vi "Change Panel.vi"(8 "error in (no error)":errorcluster, 10 "New Panel":refnum<class "Panel.lvclass">, 11 "Panel Actor in":refnum<class "Panel Actor.lvclass">) -> (0 "error out":errorcluster, 3 "Panel Actor out":refnum<class "Panel Actor.lvclass">)   [LabVIEW 2017, in "MGI-Panel Actor.lvlib" / "Panel Actor.lvclass"]
doc: "Changes the type of panel for the panel actor.\n----\nCopyright: MGI 2018\nAuthor: Derek Trepanier"
uses:
  Panel Actor.lvclass
  panel-manager/Source/Panel/Panel.lvclass
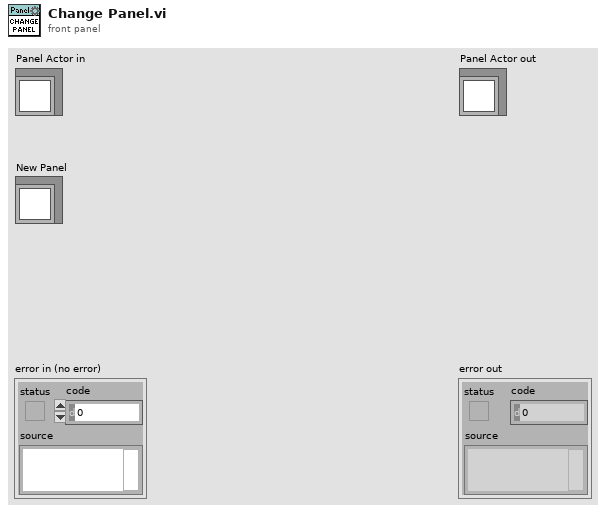
[diagram p1: front panel]
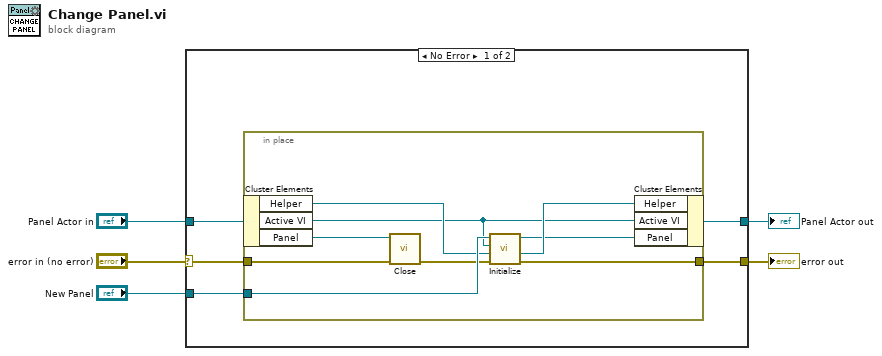
[diagram p0: block diagram]
diagram:
  n1 = case shown="No Error" "error in (no error)" {
    selector: "error in (no error)" -> [w7 w21]
    tunnel: [w6 w21] -> w4
    tunnel: [w9 w20] -> w2
    tunnel: "Panel Actor in" -> [w10 w20]
    tunnel: "New Panel" -> [w8 _]
    frame No Error {
      n2 = in-place {
        in-place-border: w8 -> [w19]
        in-place-border: w7 -> [w14]
        in-place-border: [w13] -> w6
        n3 = in-place-cluster #1(w10) -> ("Helper"=w17:refnum<class "Panel Helper.lvclass">, "Active VI"=w15:refnum<vi>, "Panel"=w11:refnum<class "Panel.lvclass">)
        n4 = call-dynamic "Close.vi"("Error In"=w14, "Panel In"=w11) -> ("Error Out"=w18:errorcluster)  [unwired: 9 in]
        n5 = call "Initialize.vi"("error in (no error)"=w18, "My Helper in"=w17, "VI Refnum"=w15, "Panel In"=w19) -> ("error out"=w13:errorcluster, "My Helper out"=w16:refnum<class "Panel Helper.lvclass">, "Panel Out"=w12:refnum<class "Panel.lvclass">)  [unwired: 5 in]
        n6 = in-place-cluster #1("Helper"=w16, "Active VI"=w15, "Panel"=w12) -> (w9:refnum<class "Panel Actor.lvclass">)
      }
    }
    frame Error {
    }
  }
  "error out" <- w4
  "Panel Actor out" <- w2
